vi "Suspend.vi"(8 "error in (no error)":errorcluster, 9 "Old data":T1={"Channels to measure"=[1.0], "Record heater"=FALSE, "Set point"=0.0, "Set Heater Range"=enum."Off", "Control"=FALSE, "Approach"=enum."Instant", "Ramp rate, K/min"=1.0, "Control Channel"=1, "P"=0.0, "I"=0.0, "D"=0.0, "Suspend heater"=FALSE}, 10 "New data":T4={"Channels to measure"=[], "Record heater"=FALSE, "Set point"=0.0, "Heater Range"=enum."25W", "Control"=FALSE, "Loop type"=enum."Off", "Ramp rate,\n K/min"=1.0, "Control Channel"="A", "P"=0.0, "I"=0.0, "D"=0.0, "Manual %"=1}, 11 "Device in":refnum<class "Cryo-Con-22C.lvclass">) -> (0 "error out":errorcluster, 3 "Device out":refnum<class "Cryo-Con-22C.lvclass">)   [LabVIEW 2015, in "Cryo-Con-22C.lvclass"]
uses:
  Cryo-Con-22C.lvclass
  Cryo-Con Front Panel Data.ctl
  Cryo-con Heater Ranges.ctl
  Cry-Con Loop Type.ctl
  Neocera/Neocera Front Panel Data.ctl
  Neocera/Neocera Heater Ranges.ctl
  Neocera/Neocera Set Point Aproach.ctl
panel:
  # "Temperature Monitor"
  # "Temperature Control"
  # "Temperature Monitor"
  # "Temperature Control"
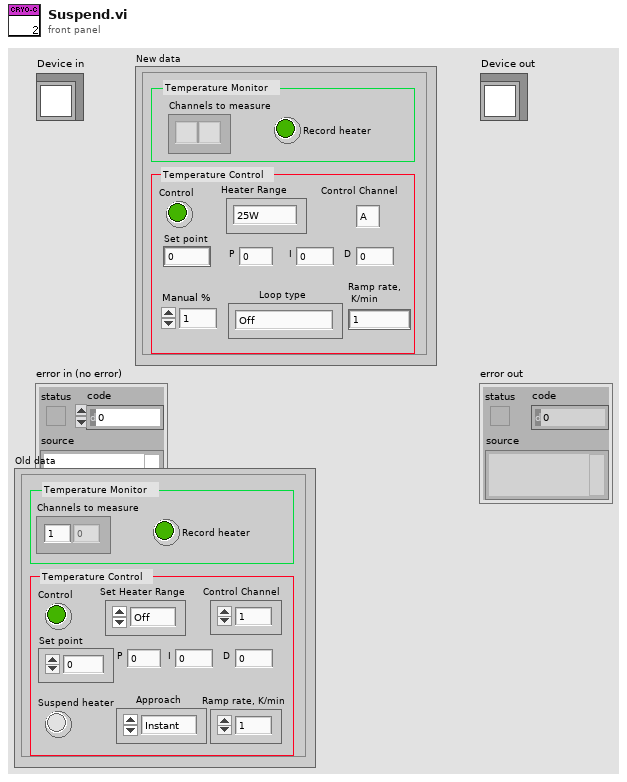
[diagram p1: front panel]
types:
  T1 = typedef "Neocera Front Panel Data.ctl" = cluster{"Channels to measure":dbl[], "Record heater":bool, "Set point":dbl, "Set Heater Range":T2, "Control":bool, "Approach":T3, "Ramp rate, K/min":dbl, "Control Channel":i16, "P":dbl, "I":dbl, "D":dbl, "Suspend heater":bool}
  T2 = typedef "Neocera Heater Ranges.ctl" = enum16{"Off", "0.05W", "0.5W", "5W", "50W"}
  T3 = typedef "Neocera Set Point Aproach.ctl" = enum16{"Instant", "Ramp"}
  T4 = typedef "Cryo-Con Front Panel Data.ctl" = cluster{"Channels to measure":string[], "Record heater":bool, "Set point":dbl, "Heater Range":T5, "Control":bool, "Loop type":T6, "Ramp rate,\n K/min":dbl, "Control Channel":string, "P":dbl, "I":dbl, "D":dbl, "Manual %":u16}
  T5 = typedef "Cryo-con Heater Ranges.ctl" = enum16{"25W", "2.5W", "0.25W"}
  T6 = typedef "Cry-Con Loop Type.ctl" = enum16{"Off", "PID", "Manual", "PID Table", "PID Ramp", "PID Table Ramp"}
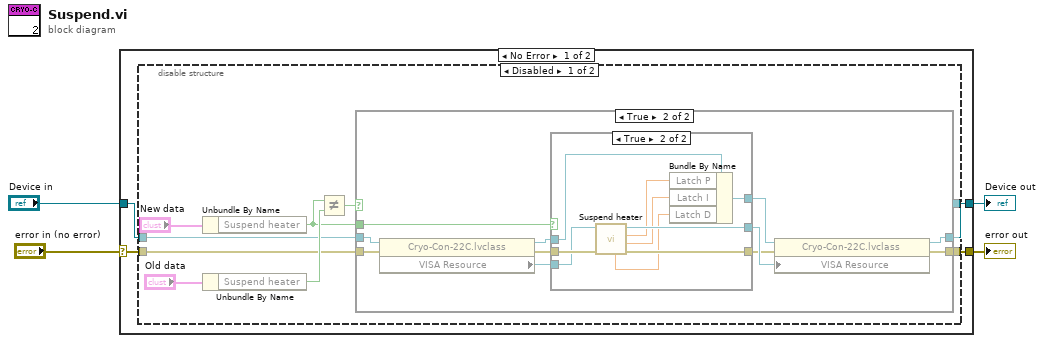
[diagram p0: block diagram]
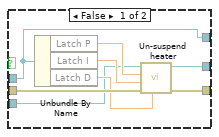
[diagram p3: hidden frame]
diagram:
  n1 = case shown="No Error" "error in (no error)" {
    selector: "error in (no error)" -> [w5 w51]
    tunnel: [w8 w51] -> w3
    tunnel: [w6 w50] -> w1
    tunnel: "Device in" -> [w7 w50]
    frame No Error {
      n2 = disable-structure shown="Disabled" {
        disable-tunnel: [w12 w48] -> w8
        disable-tunnel: w7 -> [w11 w49]
        disable-tunnel: [w10 w49] -> w6
        disable-tunnel: w5 -> [w9 w48]
        frame Disabled {
          n3 = Unbundle By Name("New data") -> ("Suspend heater"=w13:bool)
          n4 = Unbundle By Name("Old data") -> ("Suspend heater"=w15:bool)
          n5 = Not Equal?(x=w13, y=w15) -> (x != y?=w14:bool)
          n6 = case shown="True" w14 {
            tunnel: w9 -> [w19 w23]
            tunnel: [w19 w20] -> w12
            tunnel: w13 -> [_ w30]
            tunnel: w11 -> [w18 w27]
            tunnel: [w18 w26] -> w10
            frame False {
            }
            frame True {
              n7 = property class="Cryo-Con-22C.lvclass"(reference=w27, error in=w23) -> (reference out=w28:refnum<class "Cryo-Con-22C.lvclass">, error out=w22:errorcluster, "VISA Resource"=w24:refnum<visa-resource-name>)
              n8 = case shown="True" w30 {
                tunnel: [w38 w47] -> w25
                tunnel: w22 -> [w37 w46]
                tunnel: [w36 w45] -> w21
                tunnel: w28 -> [w32 w44]
                tunnel: [w32 w40] -> w29
                tunnel: w24 -> [w31 w39]
                frame False {
                  n9 = Unbundle By Name(w32) -> ("Latch P"=w35:dbl, "Latch I"=w34:dbl, "Latch D"=w33:dbl)
                  n10 = call "Un-suspend heater.vi"("D"=w33, "error in (no error)"=w37, "I"=w34, "P"=w35, "VISA Refnum in"=w31) -> ("error out"=w36:errorcluster, "VISA Refnum out"=w38:refnum<visa-resource-name>)  [unwired: 5 in]
                }
                frame True {
                  n11 = call "Suspend heater.vi"("error in (no error)"=w46, "VISA resource name"=w39) -> ("error out"=w45:errorcluster, "I"=w42:dbl, "P"=w43:dbl, "VISA resource name out"=w47:refnum<visa-resource-name>, "D"=w41:dbl)  [unwired: 4 in, 1 out]
                  n12 = Bundle By Name(cluster=w44, "Latch P"=w43, "Latch I"=w42, "Latch D"=w41) -> (w40:refnum<class "Cryo-Con-22C.lvclass">)
                }
              }
              n13 = property class="Cryo-Con-22C.lvclass"(reference=w29, error in=w21, "VISA Resource"=w25) -> (reference out=w26:refnum<class "Cryo-Con-22C.lvclass">, error out=w20:errorcluster)
            }
          }
        }
        frame Enabled {
        }
      }
    }
    frame Error {
    }
  }
  "error out" <- w3
  "Device out" <- w1
